vi "Get service UUID.vi"(8 "Error In":errorcluster, 10 "service_info":u8[][](array[numeric])) -> (0 "Error Out":errorcluster, 2 "Service UUID list":string[](array[string]))   [LabVIEW 2016]
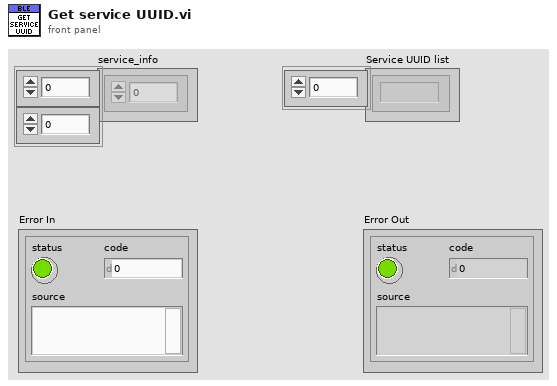
[diagram p1: front panel]
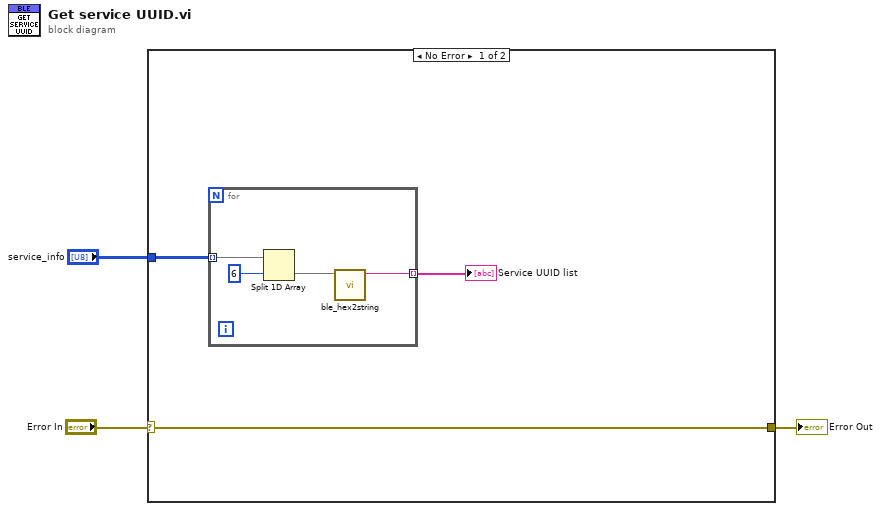
[diagram p0: block diagram]
diagram:
  n1 = case shown="No Error" "Error In" {
    selector: "Error In" -> [w6 w11]
    tunnel: [w6 w11] -> w2
    tunnel: "service_info" -> [w4 _]
    frame No Error {
      n2 = for {
        tunnel: [w10] -> w5 mode=indexing
        tunnel: w4 -> [w7] mode=indexing
        n3 = Split 1D Array(array=w7, index=6) -> (second subarray=w8:u8[])  [unwired: 1 out]
        n4 = call <vilib>:"ble_hex2string.vi"("Byte Array IN (index0 LS byte)"=w8) -> ("HEX string OUT"=w10:string)  [unwired: 10 in]
      }
      "Service UUID list" <- w5
    }
    frame Error {
    }
  }
  "Error Out" <- w2
